vi "Light Ring TestCode.vi"(10 "Step Text":string="String") -> (2 "Light Ring Output":string)   [LabVIEW 2014]
uses:
  <vilib>/Rock Robotics/WPI/Relay/WPI_RelayValue.ctl
panel:
  in  "RelayValue":T1
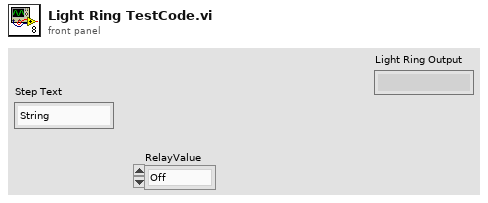
[diagram p1: front panel]
types:
  T1 = typedef "WPI_RelayValue.ctl" = enum16{"Off", "On", "Forward", "Reverse"}
  T2 = typedef "WPI_RelayDevRef.ctl" = cluster{"DevStatus":errorcluster, "Relay Channel":T3, "Controller":T4, "Relay Direction":T5}
  T3 = typedef "FPGA_DIORelayChannel.ctl" = enum8{"Relay 0", "Relay 1", "Relay 2", "Relay 3", "Invalid"}
  T4 = typedef "FPGA_TypedefDigitalModule.ctl" = enum16{"Controller 1"}
  T5 = typedef "WPI_RelayDirection.ctl" = enum16{"Both directions", "Forward only", "Reverse only"}
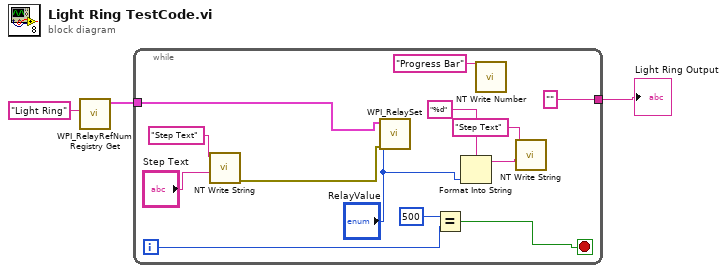
[diagram p0: block diagram]
diagram:
  n1 = call <vilib>:"WPI_RelayRefNum Registry Get.vi"("refnum name"="Light Ring") -> ("RelayDevRef"=w1:T2)  [unwired: 9 in, 1 out]
  n2 = while {
    tunnel: ["" ("Light Ring Output")] -> w3
    tunnel: w1 -> [w14]
    i -> [w12]
    stop <- w10 stop-if-true
    n3 = call <vilib>:"NT Write String.vi"("String"="Step Text", "Name"="Step Text" ("String")) -> ("error out"=w16:errorcluster)  [unwired: 9 in]
    n4 = call <vilib>:"WPI_RelaySet.vi"("error in (no error)"=w16, "RelayValue"="RelayValue", "RelayDevRef"=w14) -> ()  [unwired: 7 in, 2 out]
    n5 = Equal?(x=500, y=w12) -> (x = y?=w10:bool)
    n6 = Format Into String(format string="%d", "RelayValue") -> (resulting string=w6:string)  [unwired: 2 in, 1 out]
    n7 = call <vilib>:"NT Write Number.vi"("Name"="Progress Bar") -> ()  [unwired: 10 in, 1 out]
    n8 = call <vilib>:"NT Write String.vi"("String"=w6, "Name"="Step Text") -> ()  [unwired: 9 in, 1 out]
  }
  "Light Ring Output" <- w3
